vi "KRASS Hiport_control.vi"(0 "MyIndex":u8, 2 "command":string="SALL 03,IR,500,0,1,0.5,1,0,0", 3 "error in (no error)":errorcluster) -> (4 "CommandFB":string, 5 "Report":string, 6 "Curretn":dbl, 7 "Resistent":string, 8 "Result &Command Check":bool, 9 "error out":errorcluster={"status"=TRUE, "code"=-1073807343, "source"="VISA Configure Serial Port (Instr).vi->Intial_Hiport.vi->Hiport_driver.vi->TST_SEQ_Hiport Test.vi中的属性节点 (arg 1)"})   [LabVIEW 2015]
uses:
  <vilib>/Instr/_visa.llb/VISA Flush IO Buffer Mask.ctl
panel:
  out "CommandList":string[](array[string])=["SALL 01", "DCW", "1.70", "7500", "0", "1.0", "1.0", "0.0", "0", "0", "1.0", "0.0", "0.50", "0"]
  out "Result":bool
  out "SALL?":string[](array[string])=["SALL 01", "DCW", "1.70", "7500", "0.0", "1.0", "1.0", "0.0", "0", "0", "1.00", "0.00", "0.50", "0"]
  # "DCW Voltage 1.50kV\nMax Lmt (Current) 5000mA\nMin Lmt (Current) 0.0mA\nRamp UP 0.1s\nDwell 1.0s\nRamp DN 0.0s\nArc Sense 0\nContinuity OFF\nMax Lmt (Continuity) 1.00W\nMin Lmt (Continuity) 0.00W\nOffset (Continuity) 0.5W\nConnect OFF"
  # "[Solarcity production line hipot]"
  # "SALL 01,DCW,1.50,5000,0,1.0,1.0,1.0,0,0,1.0,0.0,0.50,0"
  # "SALL 02,ACW,2.22,3000,0,3.0,3.0,3.0,0,60,0,1.0,0.0,0.50,0"
  # "[KRASS hipot]"
  # "SALL 01,DCW,0.01,3000,0,1,1,1,0,0,0,0"
  # "SALL 02,ACW,0.2,3000,0,1,1,1,0,60,0,0"
  # "SALL 03,IR,30,0,2,1,1,1,0\n指IR模式下，电压30V, 最大阻抗不限制，最低阻抗2M欧，其余为时间和不连续"
  # "M0-3 ,IR,Pass,499V,>10G,1.0s"
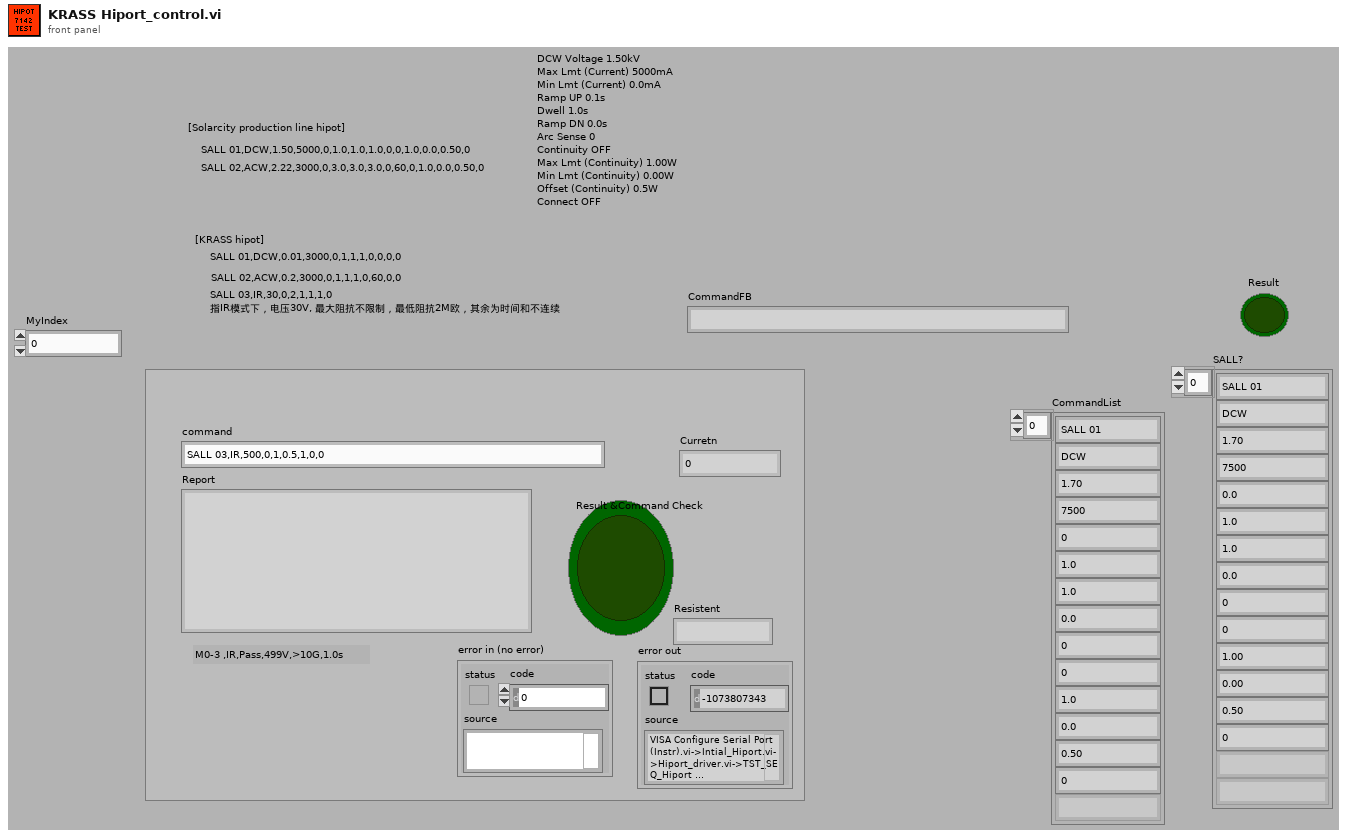
[diagram p1: front panel]
types:
  T1 = typedef "VISA Flush IO Buffer Mask.ctl" = u16
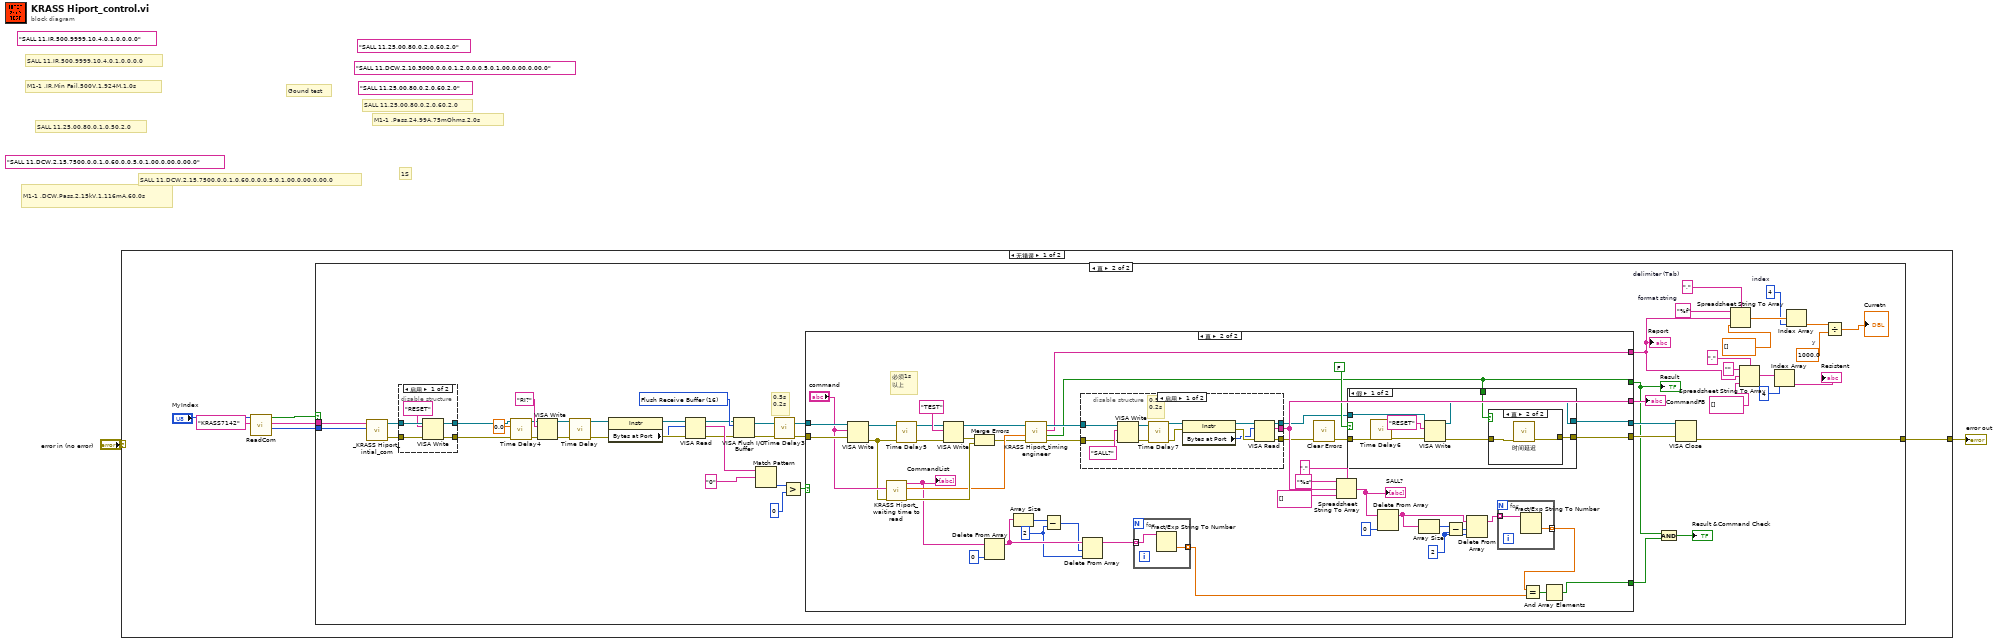
[diagram p0: block diagram]
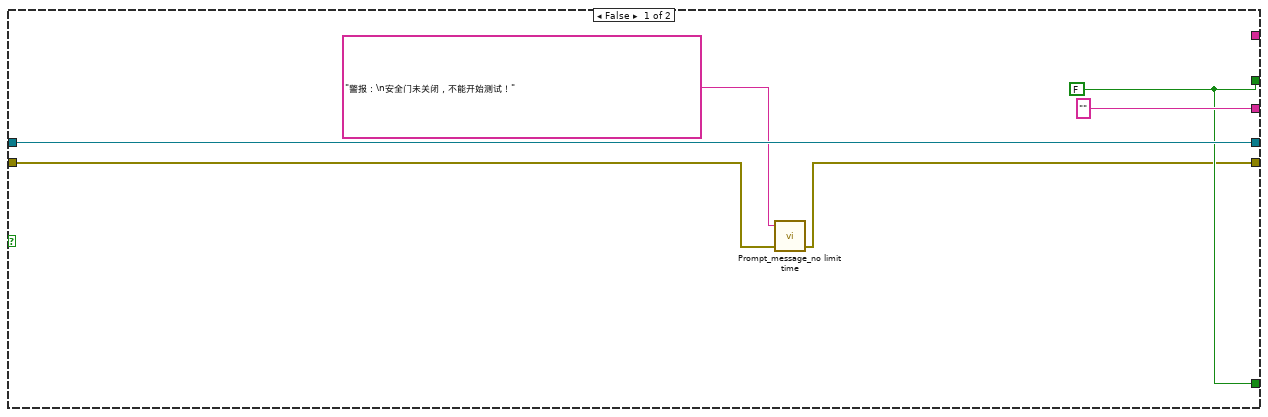
[diagram p4: hidden frame]
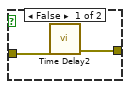
[diagram p6: hidden frame]
diagram:
  (unwired) "SALL 11,25.00,80,0,2.0,60,2,0" ("write buffer")
  (unwired) "SALL 11,25.00,80,0,2.0,60,2,0" ("write buffer")
  (unwired) "SALL 11,IR,500,9999,10,4.0,1.0,0.0,0" ("write buffer")
  (unwired) "SALL 11,DCW,2.10,3000,0.0,0.1,2.0,0.0,5,0,1.00,0.00,0.00,0" ("write buffer")
  (unwired) "SALL 11,DCW,2.15,7500,0.0,1.0,60,0.0,5,0,1.00,0.00,0.00,0" ("write buffer")
  # "1S"
  # "SALL 11,25.00,80,0,1.0,50,2,0"
  # "M1-1 ,Pass,24.99A,75mOhms,2.0s"
  # "Gound test"
  # "SALL 11,25.00,80,0,2.0,60,2,0"
  # "M1-1 ,IR,Min Fail,500V,1.924M,1.0s"
  # "SALL 11,IR,500,9999,10,4.0,1.0,0.0,0"
  # "M1-1 ,DCW,Pass,2.15kV,1.116mA,60.0s"
  # "SALL 11,DCW,2.15,7500,0.0,1.0,60.0,0.0,5,0,1.00,0.00,0.00,0"
  n1 = case shown="无错误" "error in (no error)" {
    selector: "error in (no error)" -> [_ w146]
    tunnel: [w8 w146] -> w2
    frame No Error {
      n2 = call "ReadCom.vi"("仪器名称"="KRASS7142", "MyIndex"="MyIndex") -> ("Baudrate"=w3:i32, "COM"=w5:string, "OK?"=w4:bool)  [unwired: 7 in]
      n3 = case shown="真" w4 {
        tunnel: [_ w36] -> w8
        tunnel: w5 -> [_ w10]
        tunnel: w3 -> [_ w9]
        frame False {
        }
        frame True {
          w22 = 1000.0  # y
          w24 = 4  # index
          w26 = ","  # delimiter (Tab)
          w28 = "%f"  # format string
          w44 = T1 16 items=["Flush Receive Buffer"=16, "Write Transmit Buffer to Device"=32, "Flush Receive Buffer (No I/O)"=64, "Flush Transmit Buffer"=128] ("Mask")
          # "0.5s\n0.2s"
          n4 = call "_KRASS Hiport_intial_com.vi"("baud rate"=w9, "VISA resource name"=w10) -> ("error out"=w11:errorcluster, "VISA resource name out"=w12:refnum<visa-resource-name>)  [unwired: 3 in]
          n5 = disable-structure shown="启用" {
            disable-tunnel: w12 -> [w61 w63]
            disable-tunnel: w11 -> [w60 w62]
            disable-tunnel: [w58 w63] -> w33
            disable-tunnel: [w57 w62] -> w32
            frame Enabled {
              n6 = VISA Write(VISA resource name=w61, write buffer="RESET", error in (no error)=w60) -> (VISA resource name out=w58:refnum<visa-resource-name>, error out=w57:errorcluster)  [unwired: 1 out]
            }
            frame Disabled {
            }
          }
          n7 = call "Time Delay4"("error in (no error)"=w32, "Delay Time (s)"=0.0) -> ("error out"=w35:errorcluster)  [unwired: 9 in]
          n8 = VISA Write(VISA resource name=w33, write buffer="RI?", error in (no error)=w35) -> (VISA resource name out=w56:refnum<visa-resource-name>, error out=w55:errorcluster)  [unwired: 1 out]
          n9 = call "Time Delay"("error in (no error)"=w55) -> ("error out"=w54:errorcluster)  [unwired: 10 in]
          n10 = property class="Instr"(reference=w56, error in=w54) -> (reference out=w52:refnum<visa-resource-name>, error out=w51:errorcluster, "Bytes at Port"=w50:u32)
          n11 = VISA Read(VISA resource name=w52, byte count=w50, error in (no error)=w51) -> (VISA resource name out=w43:refnum<visa-resource-name>, read buffer=w49:string, error out=w42:errorcluster)  [unwired: 1 out]
          n12 = VISA Flush I/O Buffer(VISA resource name=w43, mask (16)=w44, error in (no error)=w42) -> (VISA resource name out=w40:refnum<visa-resource-name>, error out=w41:errorcluster)
          n13 = Match Pattern(string=w49, regular expression="0") -> (offset past match=w47:i32)  [unwired: 1 in, 3 out]
          n14 = call "Time Delay3"("error in (no error)"=w41) -> ("error out"=w45:errorcluster)  [unwired: 10 in]
          n15 = Greater?(x=w47, y=0) -> (0:w37:bool)
          n16 = case shown="真" w37 {
            tunnel: w45 -> [w65 w113]
            tunnel: w40 -> [w69 w112]
            tunnel: [w69 w89] -> w39
            tunnel: [w64 w90] -> w38
            tunnel: [w67 w72] -> w31
            tunnel: [_ w92] -> w18
            tunnel: ["" ("read buffer") w91] -> w34
            tunnel: [w67 w74] -> w30
            frame False {
              w67 = FALSE
              n17 = call "Prompt_message_no limit time.vi"("error in"=w65, "Message"="警报：\n安全门未关闭，不能开始测试！") -> ("error out"=w64:errorcluster)  [unwired: 1 in, 2 out]
            }
            frame True {
              w82 = 2
              w84 = 2
              # "必须1s\n以上"
              n18 = VISA Write(VISA resource name=w112, write buffer="command", error in (no error)=w113) -> (VISA resource name out=w103:refnum<visa-resource-name>, error out=w102:errorcluster)  [unwired: 1 out]
              n19 = call "KRASS Hiport_waiting time to read.vi"("error in (no error)"=w102, "spreadsheet string"="command") -> ("error out"=w104:errorcluster, "Numeric"=w101:dbl, "CommandList"=w96:string[])  [unwired: 7 in]
              "CommandList" <- w96
              n20 = call "Time Delay5"("error in (no error)"=w102) -> ("error out"=w111:errorcluster)  [unwired: 10 in]
              n21 = VISA Write(VISA resource name=w103, write buffer="TEST", error in (no error)=w111) -> (VISA resource name out=w99:refnum<visa-resource-name>, error out=w105:errorcluster)  [unwired: 1 out]
              n22 = Merge Errors(w105, w104) -> (w100:errorcluster)
              n23 = Delete From Array(array=w96, index=0) -> (array with subset deleted=w87:string[])  [unwired: 1 in, 1 out]
              n24 = Array Size(array=w87) -> (size(s)=w86:i32)
              n25 = call "KRASS Hiport_timing engineer.vi"("error in (no error)"=w100, "WaitTime"=w101, "VISA resource name"=w99) -> ("error in (no error) 2"=w97:errorcluster, "Result"=w72:bool, "Report"=w92:string, "VISA resource name out"=w98:refnum<visa-resource-name>)  [unwired: 5 in]
              n26 = Subtract(x=w86, y=w84) -> (x-y=w85:i32)
              n27 = disable-structure shown="启用" {
                disable-tunnel: w98 -> [w119 w127]
                disable-tunnel: w97 -> [w118 w126]
                disable-tunnel: [w117 _] -> w91
                disable-tunnel: [w116 w126] -> w88
                disable-tunnel: [w114 w127] -> w70
                frame Enabled {
                  # "0.5s\n0.2s"
                  n28 = VISA Write(VISA resource name=w119, write buffer="SALL?", error in (no error)=w118) -> (VISA resource name out=w123:refnum<visa-resource-name>, error out=w121:errorcluster)  [unwired: 1 out]
                  n29 = call "Time Delay7"("error in (no error)"=w121) -> ("error out"=w122:errorcluster)  [unwired: 10 in]
                  n30 = property class="Instr"(reference=w123, error in=w122) -> (reference out=w124:refnum<visa-resource-name>, error out=w125:errorcluster, "Bytes at Port"=w115:u32)
                  n31 = VISA Read(VISA resource name=w124, byte count=w115, error in (no error)=w125) -> (VISA resource name out=w114:refnum<visa-resource-name>, read buffer=w117:string, error out=w116:errorcluster)  [unwired: 1 out]
                }
                frame Disabled {
                }
              }
              n32 = Delete From Array(array=w87, length=w85, index=w84) -> (array with subset deleted=w83:string[])  [unwired: 1 out]
              n33 = for {
                tunnel: w83 -> [w131] mode=indexing
                tunnel: [w130] -> w77 mode=indexing
                n34 = Fract/Exp String To Number(string=w131) -> (number=w130:dbl)  [unwired: 3 in, 1 out]
              }
              n35 = call <vilib>:"Clear Errors.vi"("error in (no error)"=w88) -> ("error out"=w71:errorcluster)  [unwired: 5 in, 1 out]
              n36 = Spreadsheet String To Array(delimiter (Tab)=",", format string="%s", spreadsheet string=w91, array type (2D Dbl)=string[] []) -> (array=w94:string[])
              "SALL?" <- w94
              n37 = case shown="假" FALSE {
                tunnel: w70 -> [w139 w144]
                tunnel: w71 -> [w138 w145]
                tunnel: [w133 w145] -> w90
                tunnel: [w136 w144] -> w89
                tunnel: w72 -> [w132 _]
                frame False {
                  n38 = call "Time Delay6"("error in (no error)"=w138) -> ("error out"=w135:errorcluster)  [unwired: 10 in]
                  n39 = VISA Write(VISA resource name=w139, write buffer="RESET", error in (no error)=w135) -> (VISA resource name out=w136:refnum<visa-resource-name>, error out=w137:errorcluster)  [unwired: 1 out]
                  n40 = case shown="真" w132 {
                    tunnel: w137 -> [w141 w143]
                    tunnel: [w140 w142] -> w133
                    frame False {
                      n41 = call "Time Delay2"("error in (no error)"=w141) -> ("error out"=w140:errorcluster)  [unwired: 10 in]
                    }
                    frame True {
                      n42 = call "时间延迟"("error in (no error)"=w143) -> ("error out"=w142:errorcluster)  [unwired: 10 in]
                    }
                  }
                }
                frame True {
                }
              }
              n43 = Delete From Array(array=w94, index=0) -> (array with subset deleted=w79:string[])  [unwired: 1 in, 1 out]
              n44 = Array Size(array=w79) -> (size(s)=w80:i32)
              n45 = Subtract(x=w80, y=w82) -> (x-y=w81:i32)
              n46 = Delete From Array(array=w79, length=w81, index=w82) -> (array with subset deleted=w78:string[])  [unwired: 1 out]
              n47 = for {
                tunnel: [w129] -> w76 mode=indexing
                tunnel: w78 -> [w128] mode=indexing
                n48 = Fract/Exp String To Number(string=w128) -> (number=w129:dbl)  [unwired: 3 in, 1 out]
              }
              n49 = Equal?(x=w76, y=w77) -> (x = y?=w75:bool[])
              n50 = And Array Elements(Boolean array=w75) -> (logical AND=w74:bool)
            }
          }
          "Result" <- w31
          "Report" <- w18
          "CommandFB" <- w34
          n51 = And(x=w31, y=w30) -> (x .and. y?=→"Result &Command Check":bool)
          n52 = VISA Close(VISA resource name=w39, error in (no error)=w38) -> (error out=w36:errorcluster)
          n53 = Spreadsheet String To Array(delimiter (Tab)=w26, format string=w28, spreadsheet string=w18, array type (2D Dbl)=dbl[] []) -> (array=w25:dbl[])
          n54 = Spreadsheet String To Array(delimiter (Tab)="," ("分隔符(Tab)"), format string="" ("格式字符串"), spreadsheet string=w18, array type (2D Dbl)=string[] [] ("已删除元素的数组子集")) -> (array=w16:string[])
          n55 = Index Array(array=w16, index=4 ("索引")) -> (element=→"Resistent":string)
          n56 = Index Array(array=w25, index=w24) -> (element=w23:dbl)
          n57 = Divide(x=w23, y=w22) -> (x/y=→"Curretn":dbl)
        }
      }
    }
    frame Error {
    }
  }
  "error out" <- w2
